vi "growthLaw.vi"(1 "n = Layer Number":i32, 2 "r = Height Ratio":dbl, 3 "h = Initial Height":dbl, 4 "Growth Law":string(combo)="Linear") -> (0 "Coordinates":dbl[](array[numeric]))   [LabVIEW 2013]
panel:
  out "Total Height":dbl
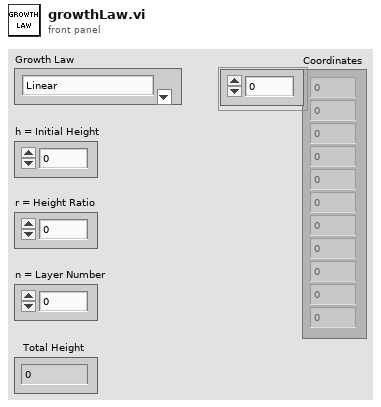
[diagram p1: front panel]
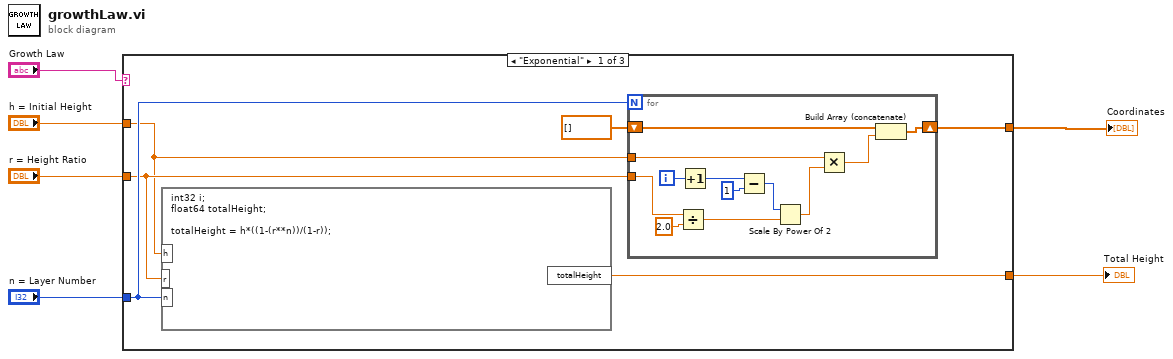
[diagram p0: block diagram]
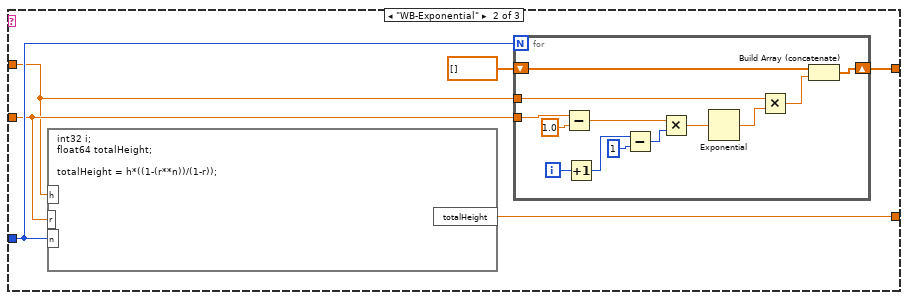
[diagram p2: hidden frame]
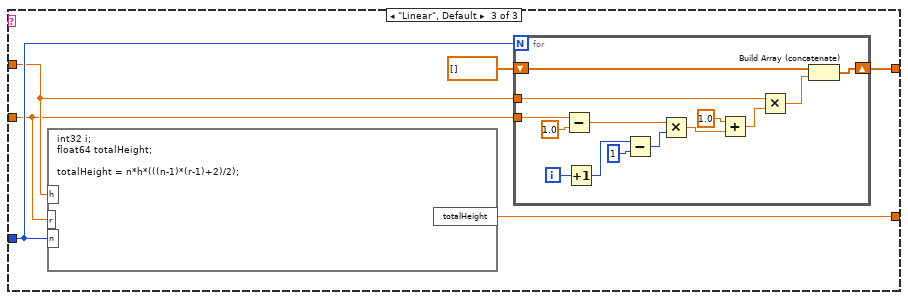
[diagram p3: hidden frame]
diagram:
  n1 = case shown="\"Exponential\"" "Growth Law" {
    tunnel: [w8 w30 w49] -> w6
    tunnel: "n = Layer Number" -> [w11 w29 w48]
    tunnel: "h = Initial Height" -> [w9 w27 w47]
    tunnel: "r = Height Ratio" -> [w10 w28 w46]
    tunnel: [w7 w25 w44] -> w1
    frame "Exponential" {
      n2 = formula code="int32 i;\nfloat64 totalHeight;\n\ntotalHeight = h*((1-(r**n))/(1-r));"("h"=w9, "r"=w10, "n"=w11) -> ("totalHeight"=w8:dbl)
      n3 = for {
        N: w11 -> [_]
        tunnel: w9 -> [w19]
        tunnel: w10 -> [w18]
        shift-right: [w21] -> w7
        shift-left: dbl[] [] -> [w20]
        i -> [w24]
        n4 = Divide(x=w18, y=2.0) -> (x/y=w16:dbl)
        n5 = Increment(x=w24) -> (x+1=w23:i32)
        n6 = Subtract(x=w23, y=1) -> (x-y=w15:i32)
        n7 = Scale By Power Of 2(n=w15, x=w16) -> (x*2^n=w14:dbl)
        n8 = Multiply(x=w19, y=w14) -> (x*y=w13:dbl)
        n9 = Build Array (concatenate)(w20, w13) -> (w21:dbl[])
      }
    }
    frame "WB-Exponential" {
      n10 = formula code="int32 i;\nfloat64 totalHeight;\n\ntotalHeight = h*((1-(r**n))/(1-r));"("h"=w27, "r"=w28, "n"=w29) -> ("totalHeight"=w30:dbl)
      n11 = for {
        N: w29 -> [_]
        tunnel: w27 -> [w38]
        tunnel: w28 -> [w36]
        shift-right: [w40] -> w25
        shift-left: dbl[] [] -> [w39]
        i -> [w43]
        n12 = Subtract(x=w36, y=1.0) -> (x-y=w34:dbl)
        n13 = Increment(x=w43) -> (x+1=w42:i32)
        n14 = Subtract(x=w42, y=1) -> (x-y=w33:i32)
        n15 = Multiply(x=w34, y=w33) -> (x*y=w32:dbl)
        n16 = Exponential(1:w32) -> (0:w31:dbl)
        n17 = Multiply(x=w38, y=w31) -> (x*y=w37:dbl)
        n18 = Build Array (concatenate)(w39, w37) -> (w40:dbl[])
      }
    }
    frame "Linear", Default {
      n19 = formula code="int32 i;\nfloat64 totalHeight;\n\ntotalHeight = n*h*(((n-1)*(r-1)+2)/2);"("h"=w47, "r"=w46, "n"=w48) -> ("totalHeight"=w49:dbl)
      n20 = for {
        N: w48 -> [_]
        tunnel: w47 -> [w62]
        tunnel: w46 -> [w58]
        shift-right: [w51] -> w44
        shift-left: dbl[] [] -> [w50]
        i -> [w63]
        n21 = Subtract(x=w58, y=1.0) -> (x-y=w56:dbl)
        n22 = Increment(x=w63) -> (x+1=w60:i32)
        n23 = Subtract(x=w60, y=1) -> (x-y=w55:i32)
        n24 = Multiply(x=w56, y=w55) -> (x*y=w54:dbl)
        n25 = Add(x=1.0, y=w54) -> (x+y=w53:dbl)
        n26 = Multiply(x=w62, y=w53) -> (x*y=w52:dbl)
        n27 = Build Array (concatenate)(w50, w52) -> (w51:dbl[])
      }
    }
  }
  "Total Height" <- w6
  "Coordinates" <- w1
